vi "Available Staffs.vi"(0 "Hotel Management Tool Model in":refnum<class "Hotel Management Tool Model.lvclass">, 5 "Staff Name":string[](array[string]), 11 "error in (no error)":errorcluster) -> (4 "Hotel Management Tool Model out":refnum<class "Hotel Management Tool Model.lvclass">, 15 "error out":errorcluster)   [LabVIEW 2023, in "Hotel Management Tool Model.lvlib" / "Hotel Management Tool Model.lvclass"]
uses:
  Hotel Management Tool Model.lvclass
  Hotel Management Tool Model.lvclass/Hotel Management Tool Model.ctl
  Room Service Monitor Model/Room Service Monitor Model Messages/Allocate Staff Msg/Allocate Staff Msg.lvclass
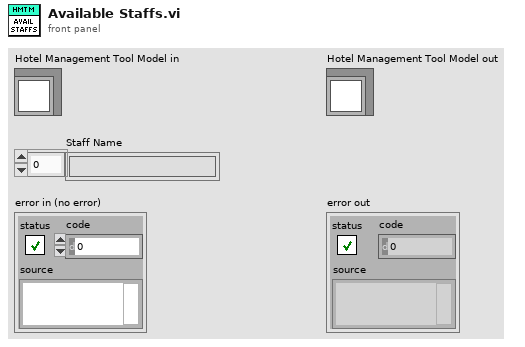
[diagram p1: front panel]
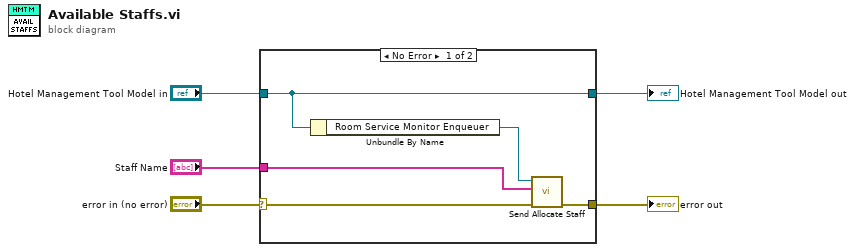
[diagram p0: block diagram]
diagram:
  n1 = case shown="No Error" "error in (no error)" {
    selector: "error in (no error)" -> [w10 w11]
    tunnel: "Hotel Management Tool Model in" -> [w9 w12]
    tunnel: [w9 w12] -> w3
    tunnel: [w8 w11] -> w2
    tunnel: "Staff Name" -> [w6 _]
    frame No Error {
      n2 = Unbundle By Name(w9) -> ("Room Service Monitor Enqueuer"=w7:refnum<class "Message Enqueuer.lvclass">)
      n3 = call "Send Allocate Staff.vi"("error in (no error)"=w10, "Staff Name"=w6, "Message Enqueuer"=w7) -> ("error out"=w8:errorcluster)  [unwired: 7 in, 1 out]
    }
    frame Error {
    }
  }
  "error out" <- w2
  "Hotel Management Tool Model out" <- w3
